vi "MercuryIPSMove.vi"(1 "Points":cluster{string, "data":u64, "data":dbl}, 2 "Inst_param":T3={"Kind"=16, "Strings"=["", "192.168.137.3", "", "GRPZ"], "uint64s"=[], "Doubles"=[-12.0, 12.0, 6.285], "DAQmx take out list"=[]}) -> ()   [LabVIEW 2013]
uses:
  <instrlib>/Mercury iXX/Public/Controls/Comms Transport Layer.ctl
  <instrlib>/Mercury iXX/Public/Controls/Serial Settings.ctl
  <instrlib>/Mercury iXX/Public/Controls/ISOBus Address.ctl
  <instrlib>/Mercury iXX/Mercury iXX.lvlib
panel:
  out "To set?":bool
  in  "Emergency stop":bool
  in  "Ramp Controls":T1={"Target Current (A)"=0.0, "Target Rate (A/min)"=0.0, "Target Field (T)"=0.0, "Target Rate (T/min)"=0.1}
  out "Status":string
  out "Mag_data":T2
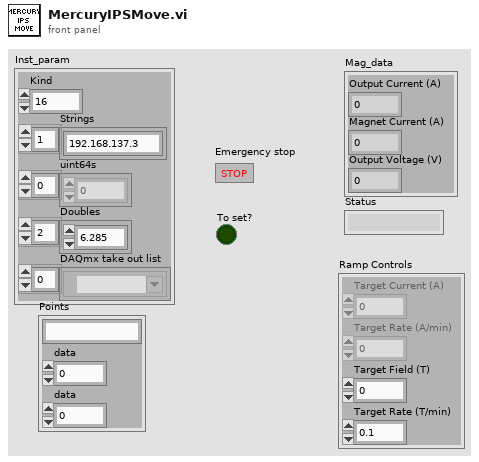
[diagram p1: front panel]
types:
  T1 = cluster{"Target Current (A)":dbl, "Target Rate (A/min)":dbl, "Target Field (T)":dbl, "Target Rate (T/min)":dbl}
  T2 = cluster{"Output Current (A)":dbl, "Magnet Current (A)":dbl, "Output Voltage (V)":dbl}
  T3 = cluster{"Kind":u16, "Strings":string[], "uint64s":u64[], "Doubles":dbl[], "DAQmx take out list":refnum<k21>[]}
  T4 = typedef "Mercury iXX.lvlib/Comms Transport Layer.ctl" = enum16{"Ethernet TCP/IP", "USB", "ISOBus - RS-232", "GPIB"}
  T5 = typedef "Mercury iXX.lvlib/Serial Settings.ctl" = cluster{"Baud Rate":u32, "Parity":u16, "Data Bits":u16, "Stop Bits":u16, "Flow Control":u16}
  T6 = typedef "Mercury iXX.lvlib/ISOBus Address.ctl" = i32
  T7 = cluster{"VISA resource name":refnum<visa-resource-name>, "Comms Layer":T4, "IP Address":string, "Serial Configuration":T5, "ISOBUS address":T6}
  T8 = cluster{"CLAMP":bool, "HOLD":bool, "TO SET":bool, "TO ZERO":bool}
  T9 = typedef "Mercury iXX.lvlib/Mercury Reference.ctl" = cluster{"Comms":refnum<visa-resource-name>, "Device ID":string[], "Comms Layer":T4, "Command":string, "Query reference":T10}
  T10 = typedef "Mercury iXX.lvlib/Query Dynamic Reference.ctl" = refnum<vi>
  T11 = cluster{"Current/Field (A/T)":dbl, "Meter_V_Lim":dbl, "Meter_I_lim":dbl}
  T12 = enum16{"Monitor", "Hold", "Clamp", "To Set", "To Zero", "Switch Heater", "Set Points"}
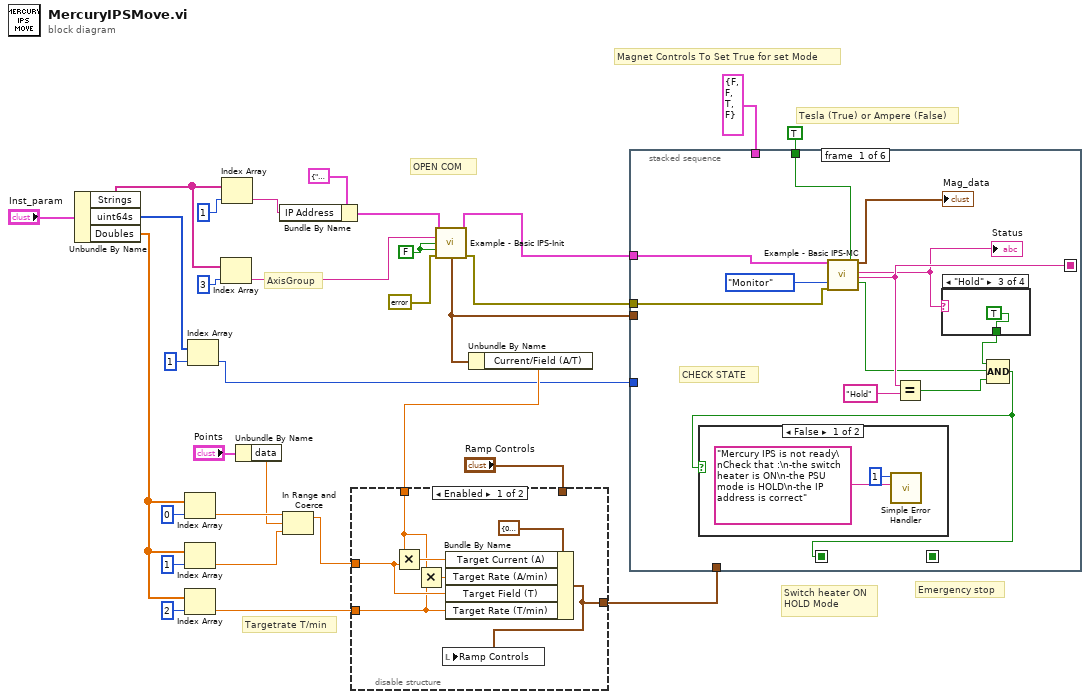
[diagram p0: block diagram]
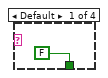
[diagram p3: hidden frame]
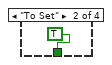
[diagram p4: hidden frame]
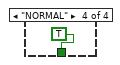
[diagram p5: hidden frame]
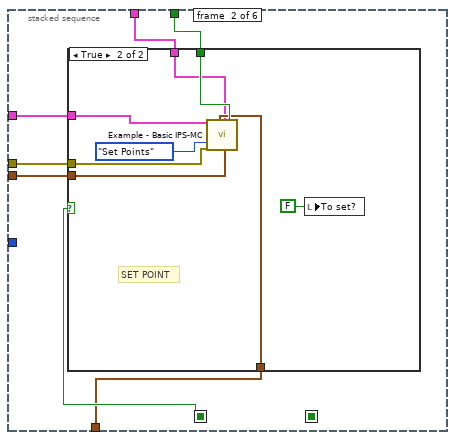
[diagram p6: hidden frame]
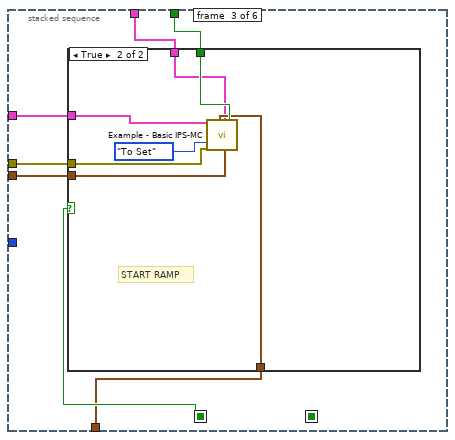
[diagram p8: hidden frame]
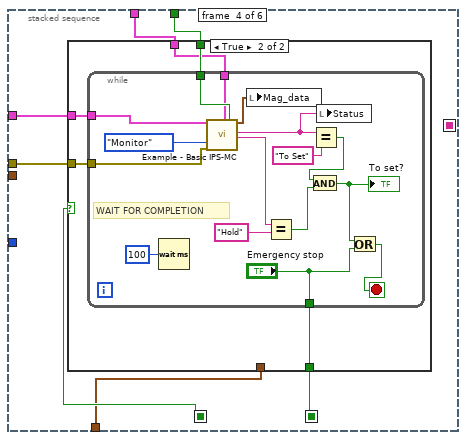
[diagram p10: hidden frame]
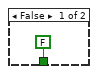
[diagram p11: hidden frame]
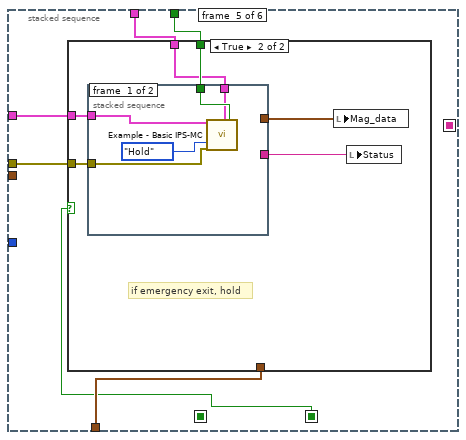
[diagram p12: hidden frame]
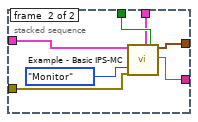
[diagram p14: hidden frame]
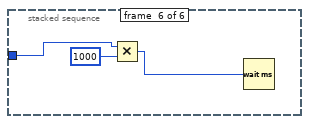
[diagram p15: hidden frame]
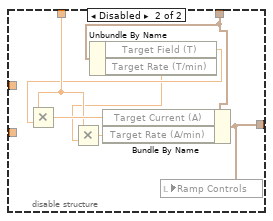
[diagram p16: hidden frame]
diagram:
  w11 = FALSE ("ID Query (True)")
  # "Emergency stop"
  # "Switch heater ON\nHOLD Mode"
  # "OPEN COM"
  # "Targetrate T/min"
  # "Magnet Controls To Set True for set Mode"
  # "Tesla (True) or Ampere (False)"
  # "AxisGroup"
  n1 = Unbundle By Name("Inst_param") -> ("Strings"=w24:string[], "uint64s"=w2:u64[], "Doubles"=w20:dbl[])
  n2 = Index Array(array=w20, index=0) -> (element=w29:dbl)
  n3 = Index Array(array=w20, index=1) -> (element=w14:dbl)
  n4 = Index Array(array=w20, index=2) -> (element=w18:dbl)
  n5 = Index Array(array=w2, index=1) -> (element=w1:u64)
  n6 = Index Array(array=w24, index=3) -> (element=w15:string)
  n7 = Index Array(array=w24, index=1) -> (element=w17:string)
  n8 = Unbundle By Name("Points") -> ("data"=w27:dbl)
  n9 = Bundle By Name(cluster=T7 {"VISA resource name"="", "Comms Layer"=enum."Ethernet TCP/IP", "IP Address"="192.168.137.3", "Serial Configuration"={"Baud Rate"=115200, "Parity"=0, "Data Bits"=8, "Stop Bits"=10, "Flow Control"=0}, "ISOBUS address"=-1} ("Connection Details"), "IP Address"=w17) -> (w16:T7)
  n10 = In Range and Coerce(upper limit=w29, x=w27, lower limit=w14) -> (coerced(x)=w19:dbl)  [unwired: 1 out]
  n11 = call <instrlib>:"Example - Basic IPS-Init.vi"("Connection Details"=w16, "Axis Group"=w15, "ID Query (True)"=w11, "Clear Previous Connections (False)"=w11, "error in (no error)"=errorcluster {"status"=FALSE, "code"=0, "source"=""}) -> ("Merc_Ref_Mag"=w4:T9, "Range_Data"=w7:T11, "error out"=w23:errorcluster)  [unwired: 1 in, 7 out]
  n12 = Unbundle By Name(w7) -> ("Current/Field (A/T)"=w6:dbl)
  n13 = disable-structure shown="Enabled" {
    disable-tunnel: w19 -> [w38 _]
    disable-tunnel: w18 -> [w34 _]
    disable-tunnel: "Ramp Controls" -> [_ w39]
    disable-tunnel: [w33 w42] -> w8
    disable-tunnel: w6 -> [w35 w43]
    frame Enabled {
      n14 = Multiply(x=w35, y=w38) -> (x*y=w37:dbl)
      n15 = Multiply(x=w35, y=w34) -> (x*y=w36:dbl)
      n16 = Bundle By Name(cluster=T1 {"Target Current (A)"=0.0, "Target Rate (A/min)"=0.0, "Target Field (T)"=0.0, "Target Rate (T/min)"=0.0} ("Ramp Controls"), "Target Current (A)"=w37, "Target Rate (A/min)"=w36, "Target Field (T)"=w38, "Target Rate (T/min)"=w34) -> (w33:T1)
      n17 = local write "Ramp Controls"(w33) -> ()
    }
    frame Disabled {
      n18 = Unbundle By Name(w39) -> ("Target Field (T)"=w41:dbl, "Target Rate (T/min)"=w40:dbl)
      n19 = Multiply(x=w43, y=w41) -> (x*y=w45:dbl)
      n20 = Multiply(x=w43, y=w40) -> (x*y=w44:dbl)
      n21 = Bundle By Name(cluster=w39, "Target Current (A)"=w45, "Target Rate (A/min)"=w44) -> (w42:T1)
      n22 = local write "Ramp Controls"(w42) -> ()
    }
  }
  n23 = stacked-sequence {
    seq-local: [w54 _ _ _ _ _] -> [_ _ _ _ _ _]
    seq-local: [w47 _ _ _ _ _] -> [_ w67 w81 w96 _ _]
    seq-local: [_ _ _ w93 _ _] -> [_ _ _ _ w122 _]
    tunnel: w23 -> [w57 w70 w85 w99 w127 _]
    tunnel: w4 -> [w55 w69 w84 w98 w126 _]
    tunnel: w7 -> [_ w64 w83 _ _ _]
    tunnel: w8 -> [_ w66 w80 w95 w124 _]
    tunnel: T8 {"CLAMP"=FALSE, "HOLD"=FALSE, "TO SET"=TRUE, "TO ZERO"=FALSE} ("Magnet Controls") -> [_ w68 w82 w97 w125 _]
    tunnel: TRUE -> [w52 w65 w79 w94 w123 _]
    tunnel: w1 -> [_ _ _ _ _ w148]
    frame #0 {
      # "CHECK STATE"
      n24 = call <instrlib>:"Example - Basic IPS-MC.vi"("Mag_Ref"=w55, "Action"=T12."Monitor", "error in (no error)"=w57, "Display Units"=w52) -> ("Mag_data"=→"Mag_data":T2, "Status"=w49:string, "Mode"=w54:string, "SW HTR\nCONFIRM"=w48:bool)  [unwired: 10 in, 2 out]
      "Status" <- w49
      n25 = Equal?(x=w54, y="Hold" ("Mode")) -> (x = y?=w53:bool)
      n26 = case shown="\"Hold\"" w49 {
        tunnel: [FALSE TRUE TRUE TRUE] -> w50
        frame Default {
        }
        frame "To Set" {
        }
        frame "Hold" {
        }
        frame "NORMAL" {
        }
      }
      n27 = Compound Arithmetic op=AND(w50, w48, w53) -> (w47:bool)
      n28 = case shown="False" w47 {
        frame False {
          n29 = call <vilib>:"Simple Error Handler.vi"("error code (no error:0)"=1, "error source (\" \")"="Mercury IPS is not ready\nCheck that :\n-the switch heater is ON\n-the PSU mode is HOLD\n-the IP address is correct" ("Mode")) -> ()  [unwired: 3 in, 5 out]
        }
        frame True {
        }
      }
    }
    frame #1 {
      n30 = case shown="True" w67 {
        tunnel: w70 -> [_ w78]
        tunnel: w69 -> [_ w76]
        tunnel: w65 -> [_ w75]
        tunnel: w68 -> [_ w73]
        tunnel: w66 -> [_ w74]
        tunnel: w64 -> [_ w71]
        frame False {
        }
        frame True {
          # "SET POINT"
          n31 = call <instrlib>:"Example - Basic IPS-MC.vi"("Mag_Ref"=w76, "Action"=T12."Set Points", "error in (no error)"=w78, "Ramp Controls"=w74, "Magnet Controls"=w73, "Range data"=w71, "Display Units"=w75) -> ()  [unwired: 7 in, 6 out]
          n32 = local write "To set?"(FALSE ("To set?")) -> ()
        }
      }
    }
    frame #2 {
      n33 = case shown="True" w81 {
        tunnel: w85 -> [_ w92]
        tunnel: w84 -> [_ w90]
        tunnel: w83 -> [_ w89]
        tunnel: w79 -> [_ w88]
        tunnel: w82 -> [_ w86]
        tunnel: w80 -> [_ w87]
        frame False {
        }
        frame True {
          # "START RAMP"
          n34 = call <instrlib>:"Example - Basic IPS-MC.vi"("Mag_Ref"=w90, "Action"=T12."To Set", "error in (no error)"=w92, "Ramp Controls"=w87, "Magnet Controls"=w86, "Range data"=w89, "Display Units"=w88) -> ()  [unwired: 7 in, 6 out]
        }
      }
    }
    frame #3 {
      n35 = case shown="True" w96 {
        tunnel: w99 -> [_ w105]
        tunnel: w98 -> [_ w104]
        tunnel: w94 -> [_ w103]
        tunnel: w97 -> [_ w102]
        tunnel: w95 -> [_ _]
        tunnel: [FALSE ("Emergency stop") w101] -> w93
        frame False {
        }
        frame True {
          n36 = while {
            tunnel: w105 -> [w121]
            tunnel: w104 -> [w119]
            tunnel: w103 -> [w118]
            tunnel: w102 -> [w117]
            tunnel: ["Emergency stop"] -> w101
            stop <- w113 stop-if-true
            # "WAIT FOR COMPLETION"
            n37 = Wait (ms)(milliseconds to wait=u32 100) -> ()  [unwired: 1 out]
            n38 = call <instrlib>:"Example - Basic IPS-MC.vi"("Mag_Ref"=w119, "Action"=T12."Monitor", "error in (no error)"=w121, "Magnet Controls"=w117, "Display Units"=w118) -> ("Mag_data"=w107:T2, "Status"=w109:string, "Mode"=w115:string)  [unwired: 9 in, 3 out]
            n39 = local write "Mag_data"(w107) -> ()
            n40 = Equal?(x=w115, y="Hold" ("Mode")) -> (x = y?=w111:bool)
            n41 = Equal?(x=w109, y="To Set" ("Mode")) -> (x = y?=w110:bool)
            n42 = And(x=w110, y=w111) -> (x .and. y?=w108:bool)
            "To set?" <- w108
            n43 = local write "Status"(w109) -> ()
            n44 = Or(x=w108, y="Emergency stop") -> (x .or. y?=w113:bool)
          }
        }
      }
    }
    frame #4 {
      n45 = case shown="True" w122 {
        tunnel: w127 -> [_ w133]
        tunnel: w126 -> [_ w132]
        tunnel: w123 -> [_ w131]
        tunnel: w125 -> [_ w130]
        tunnel: w124 -> [_ _]
        frame False {
        }
        frame True {
          # "if emergency exit, hold"
          n46 = stacked-sequence {
            tunnel: w133 -> [w138 w145]
            tunnel: w132 -> [w137 w144]
            tunnel: w131 -> [w136 w143]
            tunnel: w130 -> [w135 w142]
            tunnel: [_ w140] -> w129
            tunnel: [_ w139] -> w128
            frame #0 {
              n47 = call <instrlib>:"Example - Basic IPS-MC.vi"("Mag_Ref"=w137, "Action"=T12."Hold", "error in (no error)"=w138, "Magnet Controls"=w135, "Display Units"=w136) -> ()  [unwired: 9 in, 6 out]
            }
            frame #1 {
              n48 = call <instrlib>:"Example - Basic IPS-MC.vi"("Mag_Ref"=w144, "Action"=T12."Monitor", "error in (no error)"=w145, "Magnet Controls"=w142, "Display Units"=w143) -> ("Mag_data"=w140:T2, "Status"=w139:string)  [unwired: 9 in, 4 out]
            }
          }
          n49 = local write "Mag_data"(w129) -> ()
          n50 = local write "Status"(w128) -> ()
        }
      }
    }
    frame #5 {
      n51 = Multiply(x=w148, y=u64 1000) -> (x*y=w147:u64)
      n52 = Wait (ms)(milliseconds to wait=w147) -> ()  [unwired: 1 out]
    }
  }
